vi "DT_Find Next Triangulation_Base Point_Check.vi"(8 "left/right pt (right:F)":bool, 9 "p 3":cluster{"x":dbl, "y":dbl, "index":i32}, 10 "p 2":cluster{"x":dbl, "y":dbl, "index":i32}, 11 "p 1":cluster{"x":dbl, "y":dbl, "index":i32}) -> (1 "sin":dbl, 2 "cos":dbl, 3 "pass?":bool)   [LabVIEW 2017, in "NI_AAL_Geometry.lvlib"]
uses:
  <vilib>/Analysis/NI_AAL_Geometry.lvlib
  <vilib>/Analysis/geometry.llb/Triangle Area.vi
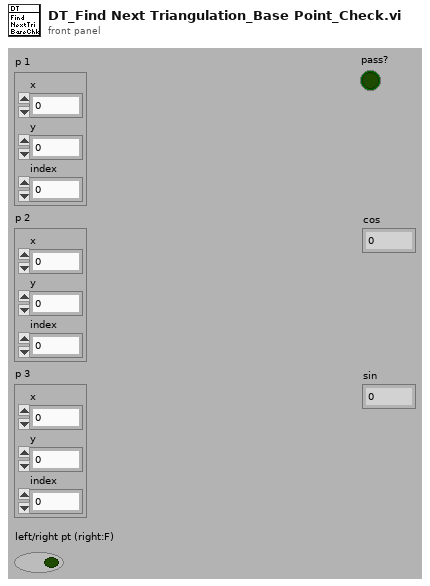
[diagram p1: front panel]
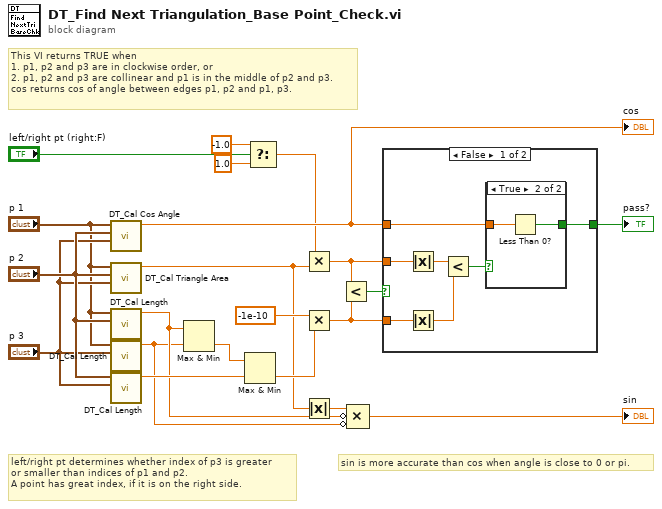
[diagram p0: block diagram]
diagram:
  # "sin is more accurate than cos when angle is close to 0 or pi."
  # "left/right pt determines whether index of p3 is greater \nor smaller than indices of p1 and p2. \nA point has great index, if it is on the right side."
  # "This VI returns TRUE when\n1. p1, p2 and p3 are in clockwise order, or\n2. p1, p2 and p3 are collinear and p1 is in the middle of p2 and p3.\ncos returns cos of angle between edges p1, p2 and p1, p3."
  n1 = call <vilib>:"DT_Cal Cos Angle.vi"("p 3"="p 3", "p 2"="p 2", "p 1"="p 1") -> ("cos"=w19:dbl)  [unwired: 8 out]
  "cos" <- w19
  n2 = call <vilib>:"DT_Cal Triangle Area.vi"("p 3"="p 3", "p 2"="p 2", "p 1"="p 1") -> ("area"=w5:dbl)  [unwired: 8 out]
  n3 = call <vilib>:"DT_Cal Length.vi"("p 2"="p 2", "p 1"="p 1") -> ("length"=w4:dbl)  [unwired: 9 out]
  n4 = call <vilib>:"DT_Cal Length.vi"("p 2"="p 3", "p 1"="p 1") -> ("length"=w3:dbl)  [unwired: 9 out]
  n5 = call <vilib>:"DT_Cal Length.vi"("p 2"="p 3", "p 1"="p 2") -> ("length"=w12:dbl)  [unwired: 9 out]
  n6 = Max & Min(x=w4, y=w3) -> (min(x,y)=w13:dbl)  [unwired: 1 out]
  n7 = Max & Min(x=w13, y=w12) -> (min(x,y)=w9:dbl)  [unwired: 1 out]
  n8 = Select(t=-1.0, s="left/right pt (right:F)", f=1.0) -> (s? t:f=w15:dbl)
  n9 = Multiply(x=w15, y=w5) -> (x*y=w14:dbl)
  n10 = Multiply(x=-1e-10 ("y"), y=w9) -> (x*y=w7:dbl)
  n11 = Absolute Value(x=w5) -> (abs(x)=w6:dbl)
  n12 = Less?(x=w14, y=w7) -> (x < y?=w21:bool)
  n13 = Compound Arithmetic op=MULTIPLY(w6, invert w4, invert w3) -> (→"sin":dbl)
  n14 = case shown="False" w21 {
    selector: w21 -> [_ w31]
    tunnel: w14 -> [w28 _]
    tunnel: [w26 w31] -> w20
    tunnel: w19 -> [w24 _]
    tunnel: w7 -> [w23 _]
    frame False {
      n15 = Absolute Value(x=w28) -> (abs(x)=w25:dbl)
      n16 = Absolute Value(x=w23) -> (abs(x)=w22:dbl)
      n17 = Less?(x=w25, y=w22) -> (x < y?=w27:bool)
      n18 = case shown="True" w27 {
        tunnel: [_ w30] -> w26
        tunnel: w24 -> [_ w29]
        frame False {
        }
        frame True {
          n19 = Less Than 0?(x=w29) -> (x < 0?=w30:bool)
        }
      }
    }
    frame True {
    }
  }
  "pass?" <- w20
